vi "Reports_GetTeamData.vi"(8 "error in (no error)":errorcluster, 11 "Refnum in":T1) -> (0 "error out":errorcluster, 2 "Array":string[][](array[string]), 3 "Refnum Out":T1)   [LabVIEW 2014, in "FIRST Reports.lvlib"]
uses:
  FIRST Reports.lvlib
  <vilib>/addons/database/Connection.llb/Conn ObjectReference.ctl
  Backend/source/VI Source/FRCts20_Backend_Engine.lvlib
  <vilib>/addons/database/NI_Database_API.lvlib
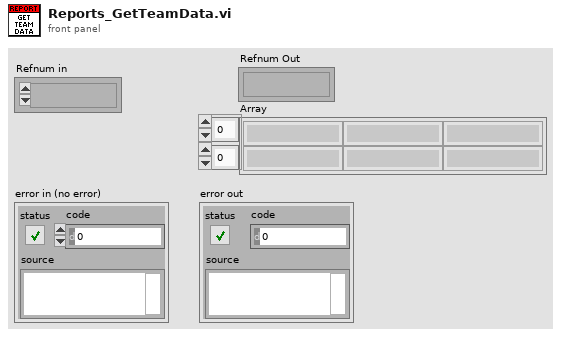
[diagram p1: front panel]
types:
  T1 = typedef "NI_Database_API.lvlib/Conn ObjectReference.ctl" = refnum<k1>
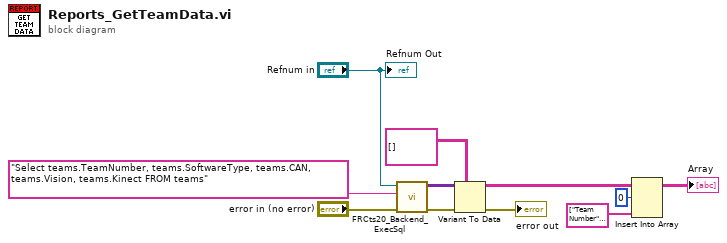
[diagram p0: block diagram]
diagram:
  n1 = call "FRCts20_Backend_ExecSql.vi"("error in (no error)"="error in (no error)", "format string"="Select teams.TeamNumber, teams.SoftwareType, teams.CAN, teams.Vision, teams.Kinect FROM teams", "Refnum in"="Refnum in") -> ("error out"=w3:errorcluster, "recordset data"=w4:variant[][])  [unwired: 6 in, 1 out]
  n2 = Variant To Data(error in=w3, type=string[][] [], Variant=w4) -> (data=w6:string[][], error out=→"error out":errorcluster)
  n3 = Insert Into Array(array=w6, index (row)=0, new element=string[] ["Team Number", "Software Type", "CAN", "Vision", "Kinect"]) -> (→"Array":string[][])  [unwired: 1 in]
  "Refnum Out" <- "Refnum in"
